vi "Uart write.vi"(0 "RedPitaya connection in":refnum<k5>, 3 "timeout ms (2000)":i32=2000, 9 "string to send":string, 11 "error in":errorcluster) -> (4 "RedPitaya connection out":refnum<k5>, 15 "error out":errorcluster)   [LabVIEW 2021]
uses:
  Variance measurement/Red_Pitaya/RedPitaya.lvlib
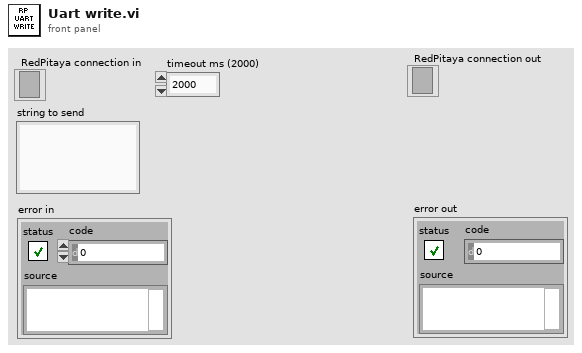
[diagram p1: front panel]
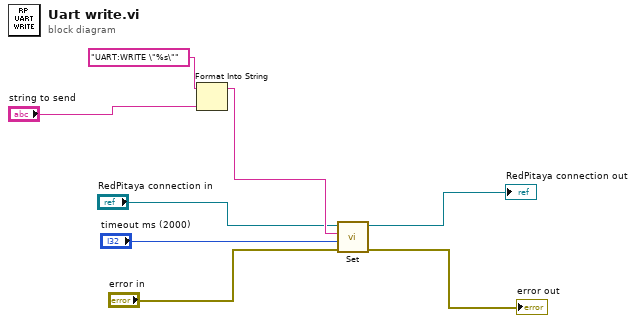
[diagram p0: block diagram]
diagram:
  n1 = Format Into String(format string="UART:WRITE \"%s\"", "string to send") -> (resulting string=w7:string)  [unwired: 2 in, 1 out]
  n2 = call "Set.vi"("error in"="error in", "timeout ms (2000)"="timeout ms (2000)", "SCPI Message"=w7, "RedPitaya connection in"="RedPitaya connection in") -> ("error out"=→"error out":errorcluster, "RedPitaya connection out"=→"RedPitaya connection out":refnum<k5>)  [unwired: 5 in, 1 out]
